vi "JSON error handler.vi"(8 "error constant":errorcluster) -> (0 "error out":errorcluster, 2 "Error?":bool, 3 "Error message out":string)   [LabVIEW 2015]
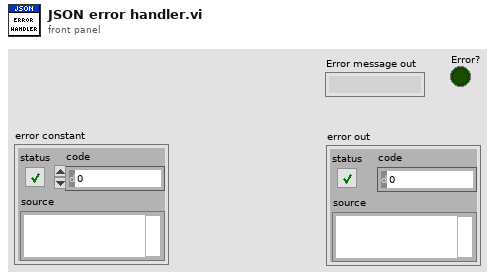
[diagram p1: front panel]
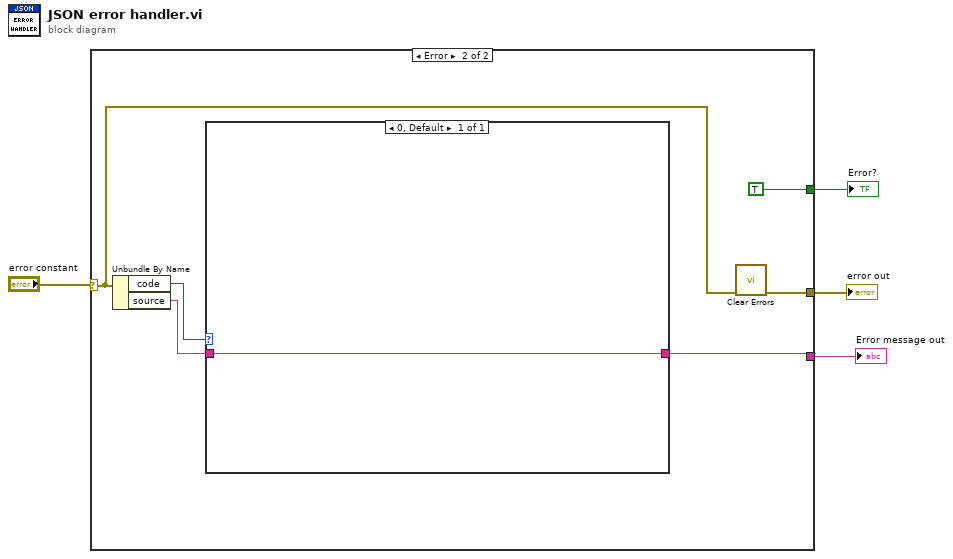
[diagram p0: block diagram]
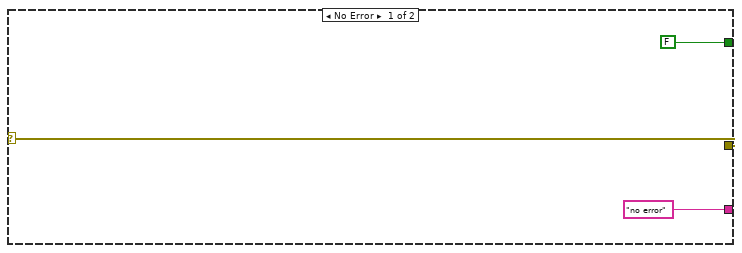
[diagram p2: hidden frame]
diagram:
  n1 = case shown="Error" "error constant" {
    selector: "error constant" -> [w7 w9]
    tunnel: ["no error" ("source") w11] -> w3
    tunnel: [w7 w10] -> w2
    tunnel: [FALSE ("Error?") TRUE ("Error?")] -> w1
    frame No Error {
    }
    frame Error {
      n2 = Unbundle By Name(w9) -> ("code"=w13:i32, "source"=w12:string)
      n3 = case shown="0, Default" w13 {
        tunnel: w12 -> [w14]
        tunnel: [w14] -> w11
        frame 0, Default {
        }
      }
      n4 = call <vilib>:"Clear Errors.vi"("error in (no error)"=w9) -> ("error out"=w10:errorcluster)  [unwired: 5 in, 1 out]
    }
  }
  "Error message out" <- w3
  "error out" <- w2
  "Error?" <- w1
